vi "PH_Sound.Device Song.vi"(3 "error in (no error)":errorcluster, 5 "Song":cluster{"Tone":dbl, "Beats":i32}[](array[cluster])) -> (0 "error out":errorcluster)   [LabVIEW 2014, in "PH_Sound.lvlib"]
uses:
  PH_Sound.lvlib
  <vilib>/sound2/lvsound2.llb/Sound Data Format.ctl
  <vilib>/sound2/lvsound2.llb/Sampling Mode.ctl
  <vilib>/sound2/lvsound2.llb/Sound Output Write (DBL Single).vi
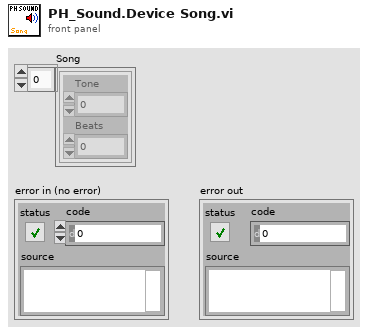
[diagram p1: front panel]
types:
  T1 = typedef "Sampling Mode.ctl" = i32
  T2 = typedef "Sound Data Format.ctl" = cluster{"sample rate (S/s)":dbl, "number of channels":i32, "bits per sample":i32}
  T3 = typedef "Sound Output Task ID.ctl" = u32
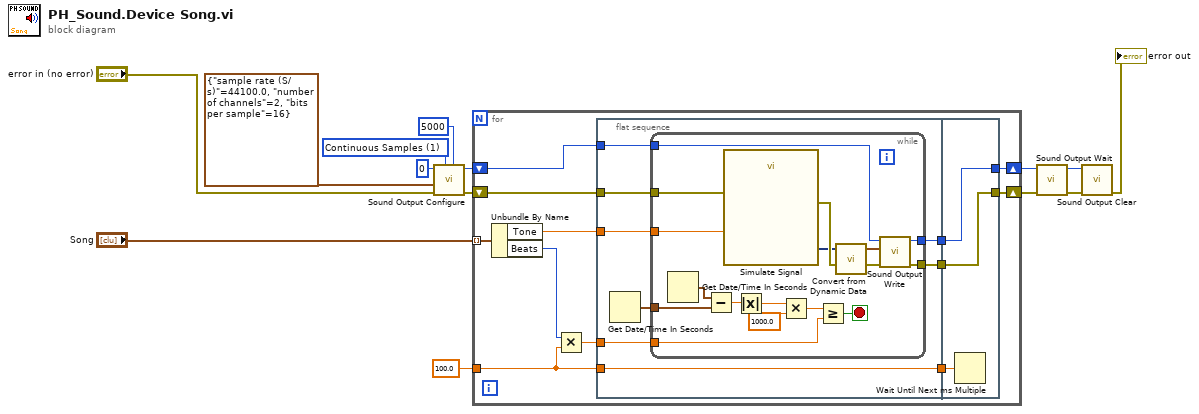
[diagram p0: block diagram]
diagram:
  w4 = T1 1 items=["Finite Samples", "Continuous Samples"] ("sample mode")
  n1 = call <vilib>:"Sound Output Configure.vi"("number of samples/ch"=5000, "sample mode"=w4, "error in (no error)"="error in (no error)", "sound format"=T2 {"sample rate (S/s)"=44100.0, "number of channels"=2, "bits per sample"=16}, "device ID"=u32 0) -> ("error out"=w9:errorcluster, "task ID"=w8:T3)  [unwired: 5 in]
  n2 = for {
    tunnel: 100.0 -> [w21]
    tunnel: "Song" -> [w25] mode=indexing
    shift-right: [w17] -> w11
    shift-left: w9 -> [w20]
    shift-right: [w15] -> w13
    shift-left: w8 -> [w19]
    n3 = Unbundle By Name(w25) -> ("Tone"=w24:dbl, "Beats"=w23:i32)
    n4 = Multiply(x=w23, y=w21) -> (x*y=w22:dbl)
    n5 = flat-sequence {
      tunnel: [w34] -> w26
      tunnel: w21 -> [w34]
      tunnel: w24 -> [w31]
      tunnel: w22 -> [w30]
      tunnel: w20 -> [w32]
      tunnel: w19 -> [w29]
      tunnel: [w28] -> w18
      tunnel: [w27] -> w16
      tunnel: w26 -> [w53]
      tunnel: w18 -> [w52]
      tunnel: [w52] -> w17
      tunnel: w16 -> [w51]
      tunnel: [w51] -> w15
      frame #0 {
        n6 = Get Date/Time In Seconds() -> (seconds since 1Jan1904=w33:timestamp)
        n7 = while {
          tunnel: w29 -> [w49]
          tunnel: w31 -> [w36]
          tunnel: w33 -> [w44]
          tunnel: w30 -> [w39]
          tunnel: w32 -> [w50]
          tunnel: [w38] -> w28
          tunnel: [w35] -> w27
          stop <- w37 stop-if-true
          n8 = Get Date/Time In Seconds() -> (seconds since 1Jan1904=w45:timestamp)
          n9 = Subtract(x=w45, y=w44) -> (x-y=w43:dbl)
          n10 = call "Simulate Signal"("Frequency"=w36, "error in (no error)"=w50) -> ("Sine"=w47:dynamicdata, "error out"=w48:errorcluster)  [unwired: 12 in]
          n11 = Absolute Value(x=w43) -> (abs(x)=w42:dbl)
          n12 = Multiply(x=w42, y=1000.0) -> (x*y=w40:dbl)
          n13 = Greater Or Equal?(x=w40, y=w39) -> (x >= y?=w37:bool)
          n14 = call "Convert from Dynamic Data"("Dynamic Data Type"=w47) -> ("Waveform"=w46:waveform(dbl))  [unwired: 3 in]
          n15 = call-poly <vilib>:"Sound Output Write.vi"("error in (no error)"=w48, "data"=w46, "task ID"=w49) -> ("error out"=w38:errorcluster, "task ID out"=w35:T3)  [unwired: 7 in]
        }
      }
      frame #1 {
        n16 = Wait Until Next ms Multiple(millisecond multiple=w53) -> ()  [unwired: 1 out]
      }
    }
  }
  n17 = call <vilib>:"Sound Output Wait.vi"("error in (no error)"=w11, "task ID"=w13) -> ("error out"=w12:errorcluster, "task ID out"=w14:T3)  [unwired: 8 in]
  n18 = call <vilib>:"Sound Output Clear.vi"("error in (no error)"=w12, "task ID"=w14) -> ("error out"=→"error out":errorcluster)  [unwired: 9 in]
